vi "Query Power On State.vi"(7 "Slave Address":i32=-1 min=-1 max=30 step=1, 8 "error":errorcluster, 11 "VISA":refnum<visa-resource-name>) -> (0 "error out":errorcluster, 2 "Power-On":enum16{"Safe-Start", "Auto-Start"}(ring), 3 "VISA out":refnum<visa-resource-name>)   [LabVIEW 2025, in "TDK-Lambda GEN LAN Series.lvlib"]
doc: "Reads the Power-On state of the power supply. The output enumerated type may be:\n\n(0) Safe Start. The power-supply will power-up with its output off. Also, after non-latching faults are cleared, the output will remain off.\n(1) Auto-Start. The power-supply will power-up in it's last state before the power was turned off. Also, after non-latching faults are cleared, the output will turn back on automatically."
uses:
  <userlib>/TDK-Lambda GEN LAN Series/TDK-Lambda GEN LAN Series.lvlib
panel:
  # "TDK-Lambda Genesys \n LAN\n  DC Power Supplies"
  # "Query Power-On State,\nSafe-Start or Auto-Start"
  # "(c) 2019 TDK-Lambda.  ALL RIGHTS RESERVED."
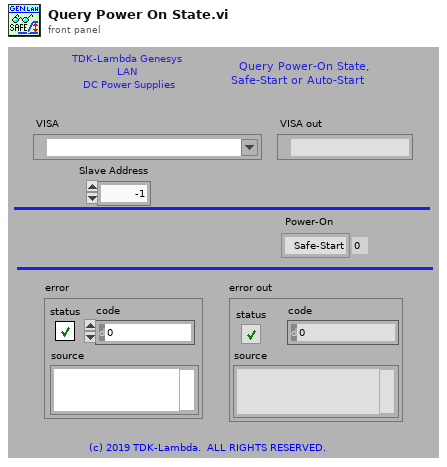
[diagram p1: front panel]
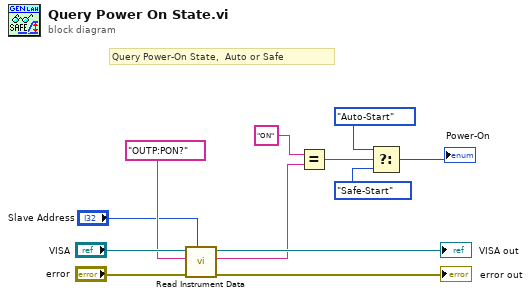
[diagram p0: block diagram]
diagram:
  # "Query Power-On State,  Auto or Safe"
  n1 = call <userlib>:"Read Instrument Data.vi"("Slave Address"="Slave Address", "error"="error", "Query"="OUTP:PON?", "VISA"="VISA") -> ("error out"=→"error out":errorcluster, "Response"=w6:string, "VISA out"=→"VISA out":refnum<visa-resource-name>)  [unwired: 4 in, 1 out]
  n2 = Equal?(x="ON", y=w6) -> (x = y?=w5:bool)
  n3 = Select(t=enum16{"Safe-Start", "Auto-Start"}."Auto-Start" ("Power-On"), s=w5, f=enum16{"Safe-Start", "Auto-Start"}."Safe-Start" ("Power-On")) -> (s? t:f=→"Power-On":enum16{"Safe-Start", "Auto-Start"})
